vi "closeneodevices.vi"(8 "error in (no error)":errorcluster, 11 "hObject":i32=1) -> (0 "error out":errorcluster, 2 "pNumberOfErrors":i32, 3 "hObject Out":i32=1)   [LabVIEW 2018]
doc: "this vi closes the port opened to the device and free the object memory\n\n<B>hObject</B> : the object reference\n\n<B>pNumberOfErrors</B> : returns the number of errors in the neoVI error queue\n\n12/21/2010 1.0.0 jyg\n- initial release"
uses:
  icsneo40.dll
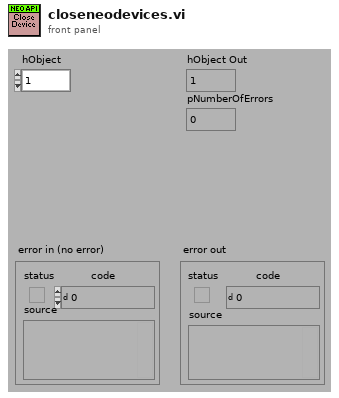
[diagram p1: front panel]
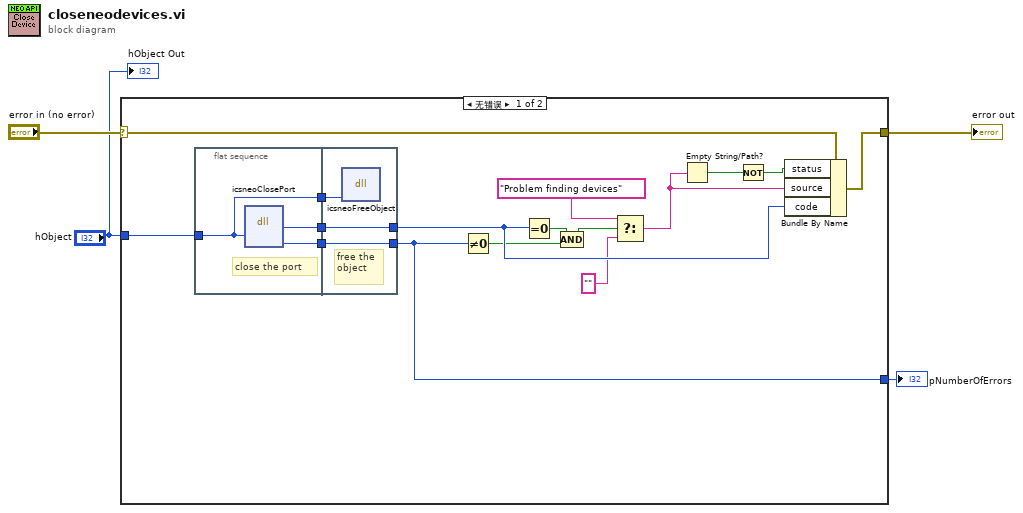
[diagram p0: block diagram]
diagram:
  n1 = case shown="无错误" "error in (no error)" {
    selector: "error in (no error)" -> [w16 w27]
    tunnel: "hObject" -> [w13 _]
    tunnel: [w17 w27] -> w4
    tunnel: [w6 _] -> w2
    frame No Error {
      n2 = flat-sequence {
        tunnel: w13 -> [w22]
        tunnel: [w23] -> w8
        tunnel: [w22] -> w7
        tunnel: [w21] -> w5
        tunnel: [w26] -> w15
        tunnel: w8 -> [w26]
        tunnel: w7 -> [w25]
        tunnel: [w24] -> w6
        tunnel: w5 -> [w24]
        frame #0 {
          # "close the port"
          n3 = dll-call lib="icsneo40.dll" fn="icsneoClosePort"("hObject"=w22) -> ("return type"=w23:i32, "pNumberOfErrors"=w21:i32)  [unwired: 4 in, 3 out]
        }
        frame #1 {
          # "free the\nobject"
          n4 = dll-call lib="icsneo40.dll" fn="icsneoFreeObject"("hObject"=w25) -> ()  [unwired: 4 in, 3 out]
        }
      }
      n5 = Not Equal To 0?(x=w6) -> (x != 0?=w11:bool)
      n6 = Equal To 0?(x=w15) -> (x = 0?=w12:bool)
      n7 = Compound Arithmetic op=AND(w12, w11) -> (w10:bool)
      n8 = Select(t="Problem finding devices", s=w10, f="") -> (s? t:f=w14:string)
      n9 = Empty String/Path?(string/path=w14) -> (empty?=w19:bool)
      n10 = Not(x=w19) -> (.not. x?=w18:bool)
      n11 = Bundle By Name(cluster=w16, "status"=w18, "source"=w14, "code"=w15) -> (w17:errorcluster)
    }
    frame Error {
    }
  }
  "error out" <- w4
  "pNumberOfErrors" <- w2
  "hObject Out" <- "hObject"
